vi "VoltageVbusConvert.vi"   [LabVIEW 2015]
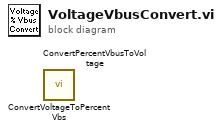
[diagram p0: block diagram]
diagram:
  n1 = call "ConvertVoltageToPercentVbs.vi"() -> ()  [unwired: 11 in, 1 out]
  n2 = call "ConvertPercentVbusToVoltage.vi"() -> ()  [unwired: 11 in, 1 out]
